vi "ReadExternalInterfaces.vi"(8 "ErrorIn":errorcluster, 11 "OpenCVFaceDetectionIn":refnum<class "OpenCVFaceDetection.lvclass">) -> (0 "ErrorOut":errorcluster, 2 "ExternalInterfaces":T1[](array[typedef]), 3 "OpenCVFaceDetectionOut":refnum<class "OpenCVFaceDetection.lvclass">)   [LabVIEW 2021, in "OpenCVFaceDetection.lvclass"]
uses:
  OpenCVFaceDetection.lvclass
  Library_TAF_Support/ClusterArrayConversion/BundledArray.ctl
  OpenCVFaceDetection.lvclass/OpenCVFaceDetection.ctl
  440278e9-1c04-4840-94c9-ed200201a6f0.vi
  Library_TAF_Support/ClusterArrayConversion/ClusterArrayConversion.lvlib
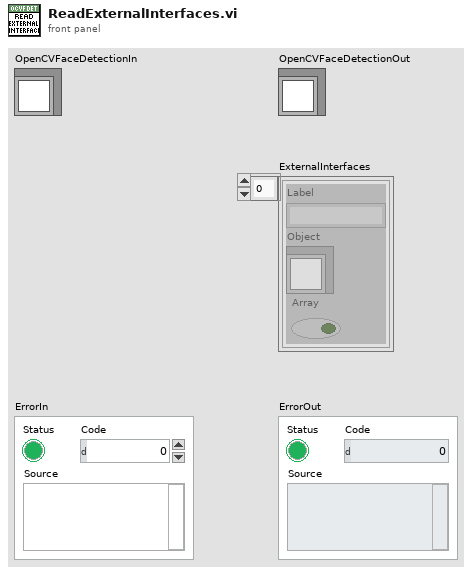
[diagram p1: front panel]
types:
  T1 = typedef "ClusterArrayConversion.lvlib/BundledArray.ctl" = cluster{"Label":string, "Object":refnum<class>, "Array":bool}
  T2 = cluster{"TAFObject":refnum<class "ITAFObject.lvclass">}
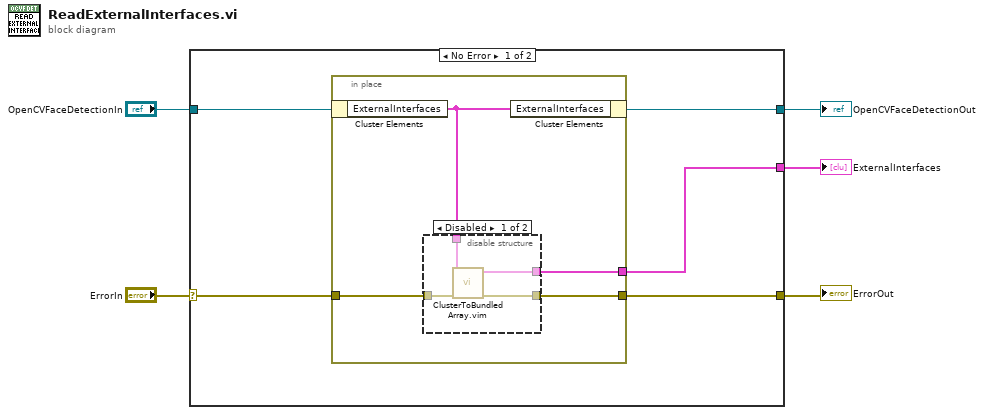
[diagram p0: block diagram]
diagram:
  n1 = case shown="No Error" "ErrorIn" {
    selector: "ErrorIn" -> [w10 w20]
    tunnel: [w9 w20] -> w4
    tunnel: [w7 w19] -> w2
    tunnel: "OpenCVFaceDetectionIn" -> [w8 w19]
    tunnel: [w6 _] -> w1
    frame No Error {
      n2 = in-place {
        in-place-border: w10 -> [w14]
        in-place-border: [w13] -> w9
        in-place-border: [w11] -> w6
        n3 = in-place-cluster #1(w8) -> ("ExternalInterfaces"=w12:T2)
        n4 = disable-structure shown="Disabled" {
          disable-tunnel: w14 -> [w18 _]
          disable-tunnel: w12 -> [w16 _]
          disable-tunnel: [w17 _] -> w13
          disable-tunnel: [w15 _] -> w11
          frame Disabled {
            n5 = call "ClusterToBundledArray.vim"("ErrorIn"=w18, "Interfaces"=w16) -> ("ErrorOut"=w17:errorcluster, "BundeledLabels"=w15:T1[])  [unwired: 8 in]
          }
          frame Enabled {
          }
        }
        n6 = in-place-cluster #1("ExternalInterfaces"=w12) -> (w7:refnum<class "OpenCVFaceDetection.lvclass">)
      }
    }
    frame Error {
    }
  }
  "ErrorOut" <- w4
  "OpenCVFaceDetectionOut" <- w2
  "ExternalInterfaces" <- w1
